vi "RemoveVimsFromProject.vi"(8 "error in (no error)":errorcluster, 11 "Project Path":path=path "C:/serenial/libraries/g-augmented-reality-toolkit/build/source-distribution/g-ar-toolkit.lvproj") -> (0 "error out":errorcluster)   [LabVIEW 2020]
uses:
  vim-liner/vim-liner.lvlib
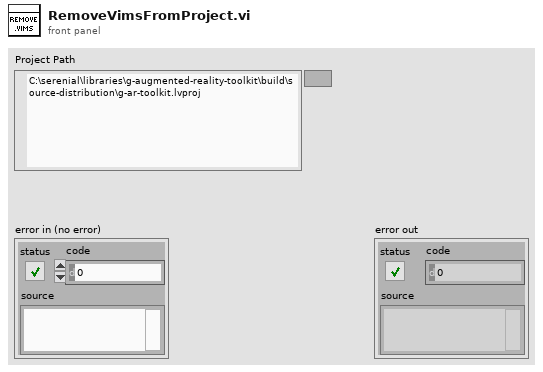
[diagram p1: front panel]
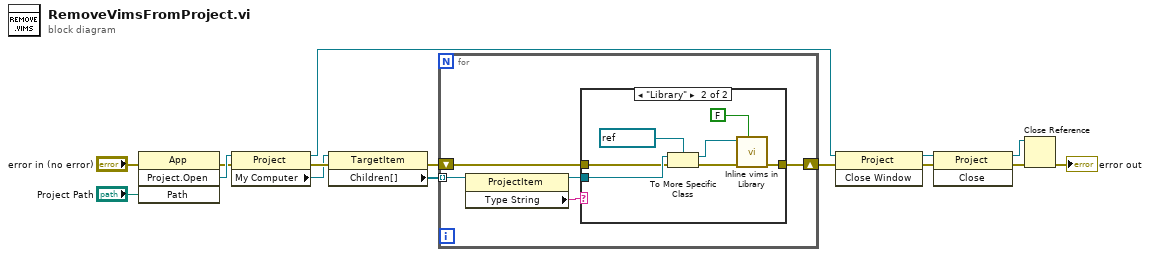
[diagram p0: block diagram]
diagram:
  n1 = invoke class="App" method="Project.Open"(error in="error in (no error)", "Path"="Project Path") -> (error out=w9:errorcluster, "Project:Open"=w10:refnum<vi>)  [unwired: 2 in, 2 out]
  n2 = property class="Project"(reference=w10, error in=w9) -> (reference out=w4:refnum<vi>, error out=w7:errorcluster, "My Computer"=w6:refnum<vi>)
  n3 = property class="TargetItem"(reference=w6, error in=w7) -> (error out=w3:errorcluster, "Children[]"=w8:refnum<vi>[])  [unwired: 1 out]
  n4 = for {
    shift-right: [w19] -> w11
    shift-left: w3 -> [w20]
    tunnel: w8 -> [w18] mode=indexing
    n5 = property class="ProjectItem"(reference=w18) -> (reference out=w16:refnum<vi>, "Type String"=w17:string)  [unwired: 1 in, 1 out]
    n6 = case shown="\"Library\"" w17 {
      tunnel: w20 -> [w21 w24]
      tunnel: [w21 w28] -> w19
      tunnel: w16 -> [_ w26]
      frame Default {
      }
      frame "Library" {
        n7 = To More Specific Class(target class=refnum<vi> refnum ("Library"), reference=w26, error in=w24) -> (specific class reference=w22:refnum<vi>, error out=w23:errorcluster)
        n8 = call "Inline vims in Library.vi"("Just Fixup"=FALSE, "error in"=w23, "Library"=w22) -> ("error out"=w28:errorcluster)  [unwired: 8 in]
      }
    }
  }
  n9 = invoke class="Project" method="Close Window"(reference=w4, error in=w11) -> (reference out=w13:refnum<vi>, error out=w15:errorcluster)  [unwired: 1 in, 1 out]
  n10 = invoke class="Project" method="Close"(reference=w13, error in=w15) -> (reference out=w12:refnum<vi>, error out=w14:errorcluster)  [unwired: 1 in, 1 out]
  n11 = Close Reference(reference=w12, error in (no error)=w14) -> (error out=→"error out":errorcluster)
